vi "Read GIF File Example.vi"(8 "error in (no error)":errorcluster, 11 "path to GIF file":path) -> (0 "error out":errorcluster, 3 "Array":u32[][](array[colorbox]))   [LabVIEW 2009]
uses:
  <vilib>/picture/picture.llb/imagedata.ctl
panel:
  out "image data":T1
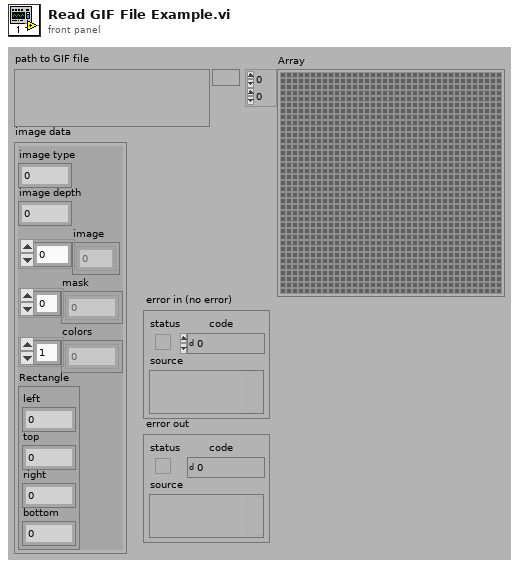
[diagram p1: front panel]
types:
  T1 = typedef "imagedata.ctl" = cluster{"image type":i32, "image depth":i32, "image":u8[], "mask":u8[], "colors":u32[], "Rectangle":cluster{"left":i16, "top":i16, "right":i16, "bottom":i16}}
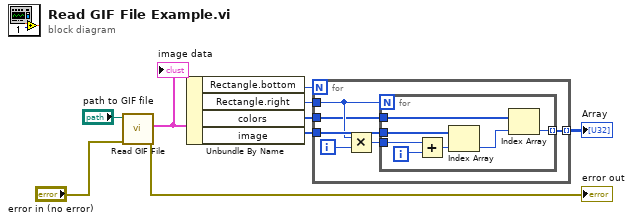
[diagram p0: block diagram]
diagram:
  n1 = call "Read GIF File.vi"("error in (no error)"="error in (no error)", "path to GIF file"="path to GIF file") -> ("error out"=→"error out":errorcluster, "image data"=w8:T1)  [unwired: 7 in, 1 out]
  "image data" <- w8
  n2 = Unbundle By Name(w8) -> ("Rectangle.bottom"=w6:i16, "Rectangle.right"=w5:i16, "colors"=w3:u32[], "image"=w4:u8[])
  n3 = for {
    N: w6 -> [_]
    tunnel: w5 -> [w13]
    tunnel: w4 -> [w15]
    tunnel: w3 -> [w11]
    tunnel: [w10] -> w7 mode=indexing
    i -> [w14]
    n4 = Multiply(x=w13, y=w14) -> (x*y=w12:i32)
    n5 = for {
      N: w13 -> [_]
      tunnel: w15 -> [w22]
      tunnel: w12 -> [w21]
      tunnel: w11 -> [w18]
      tunnel: [w16] -> w10 mode=indexing
      i -> [w20]
      n6 = Add(x=w21, y=w20) -> (x+y=w19:i32)
      n7 = Index Array(array=w22, index=w19) -> (element=w17:u8)
      n8 = Index Array(array=w18, index=w17) -> (element=w16:u32)
    }
  }
  "Array" <- w7
